vi "read shot history.vi"() -> ()   [LabVIEW 2015]
panel:
  out "String":string
  in  "File Path Control":path=path "Z:/ShotHistory2013.txt"
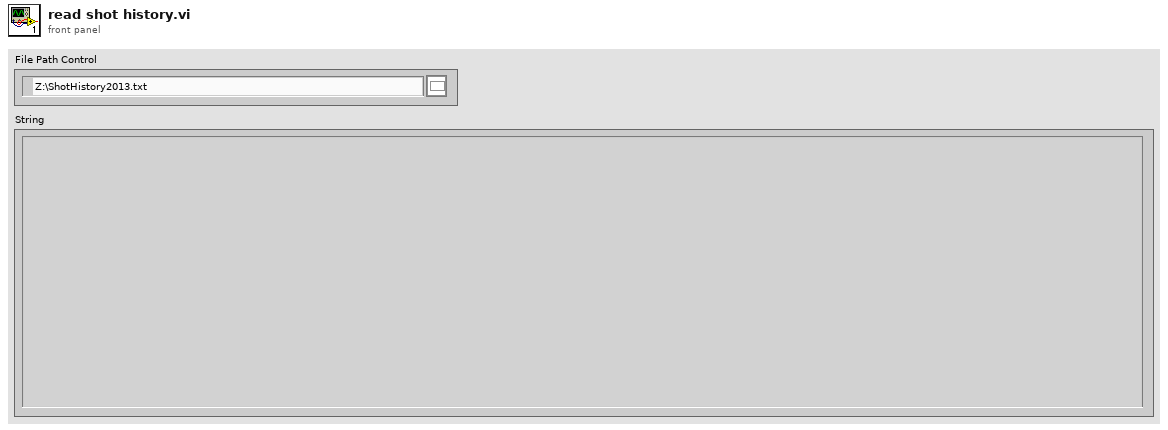
[diagram p1: front panel]
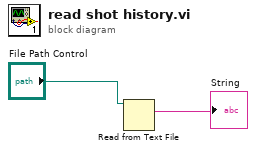
[diagram p0: block diagram]
diagram:
  n1 = Read from Text File(file (use dialog)="File Path Control") -> (text=→"String":string)  [unwired: 3 in, 3 out]
